vi "Autotune Status.vi"(8 "error in (no error)":errorcluster, 11 "VISA resource name":refnum<visa-resource-name>) -> (0 "error out":errorcluster, 1 "Tuning Error?":bool, 2 "Tuning Active?":bool, 3 "VISA resource name out":refnum<visa-resource-name>, 4 "Stage Status":u16, 5 "Output's Control Loop":u16(ring)=1 items=["1"=1, "2"=2])   [LabVIEW 2013, in "Lake Shore 336.lvlib"]
doc: "This VI returns status information on the Autotune function."
uses:
  Lake Shore 336.lvlib
  Instance           1 23Saved   Autotune Status .vi
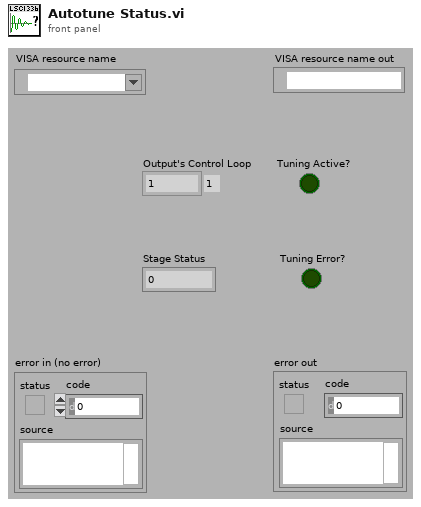
[diagram p1: front panel]
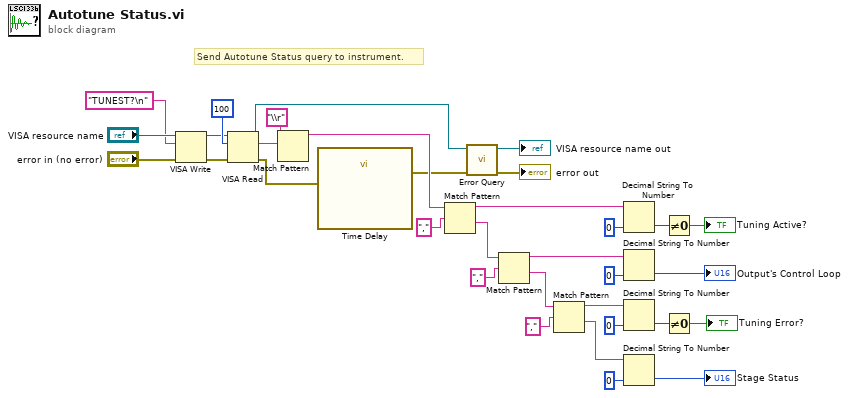
[diagram p0: block diagram]
diagram:
  # "Send Autotune Status query to instrument."
  n1 = VISA Write(VISA resource name="VISA resource name", write buffer="TUNEST?\n", error in (no error)="error in (no error)") -> (VISA resource name out=w27:refnum<visa-resource-name>, error out=w26:errorcluster)  [unwired: 1 out]
  n2 = VISA Read(VISA resource name=w27, byte count=100, error in (no error)=w26) -> (VISA resource name out=w21:refnum<visa-resource-name>, read buffer=w29:string, error out=w25:errorcluster)  [unwired: 1 out]
  n3 = Match Pattern(string=w29, regular expression="\\r") -> (before substring=w24:string)  [unwired: 1 in, 3 out]
  n4 = call "Time Delay"("error in (no error)"=w25) -> ("error out"=w20:errorcluster)  [unwired: 10 in]
  n5 = Match Pattern(string=w24, regular expression=",") -> (before substring=w10:string, after substring=w18:string)  [unwired: 1 in, 2 out]
  n6 = call "Error Query.vi"("error in (no error)"=w20, "VISA resource name"=w21) -> ("error out"=→"error out":errorcluster, "VISA resource name out"=→"VISA resource name out":refnum<visa-resource-name>)  [unwired: 7 in, 1 out]
  n7 = Match Pattern(string=w18, regular expression=",") -> (before substring=w9:string, after substring=w7:string)  [unwired: 1 in, 2 out]
  n8 = Match Pattern(string=w7, regular expression=",") -> (before substring=w6:string, after substring=w5:string)  [unwired: 1 in, 2 out]
  n9 = Decimal String To Number(string=w10, default (0L)=u16 0) -> (number=w15:u16)  [unwired: 1 in, 1 out]
  n10 = Decimal String To Number(string=w9, default (0L)=u16 0) -> (number=→"Output's Control Loop":u16)  [unwired: 1 in, 1 out]
  n11 = Decimal String To Number(string=w6, default (0L)=u16 0) -> (number=w13:u16)  [unwired: 1 in, 1 out]
  n12 = Decimal String To Number(string=w5, default (0L)=u16 0) -> (number=→"Stage Status":u16)  [unwired: 1 in, 1 out]
  n13 = Not Equal To 0?(x=w15) -> (x != 0?=→"Tuning Active?":bool)
  n14 = Not Equal To 0?(x=w13) -> (x != 0?=→"Tuning Error?":bool)
